vi "Acquisition Polling Time--constant.vi"() -> (3 "Acquisition Polling Time (ms*":i32=300)   [LabVIEW 2024, in "RaspberryPiPico.lvlib"]
uses:
  RaspberryPiPico.lvlib
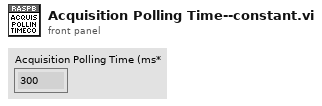
[diagram p1: front panel]
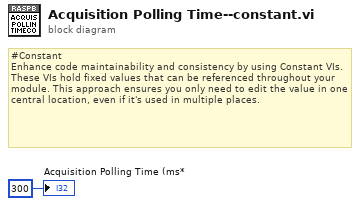
[diagram p0: block diagram]
diagram:
  # "#Constant\nEnhance code maintainability and consistency by using Constant VIs. These VIs hold fixed values that can be referenced throughout your module. This approach ensures you only need to edit the value in one central location, even if it's used in multiple places."
  "Acquisition Polling Time (ms*" <- 300 ("Acquisition Polling Time (ms*")
